vi "NI_USB.vi"() -> ()   [LabVIEW 2014]
doc: "Measure data from NI USB 6343"
uses:
  <vilib>/DAQmx/read.llb/DAQmx Read (Analog 1D Wfm NChan NSamp).vi
  <vilib>/DAQmx/configure/timing.llb/DAQmx Timing (Sample Clock).vi
  <vilib>/DAQmx/create/channels.llb/DAQmx Create Channel (AI-Voltage-Basic).vi
  <resource>/objmgr/daqmx.rc
panel:
  in  "Open PDF":bool
  in  "Help":bool
  out "Realization":dbl caption="Реализация"
  in  "Number of Samples":i16=100 caption="Буффер, от." min=10 max=2000 step=1
  out "init":bool
  in  "Sample Rate":dbl=1000.0 caption="Частота дискретизации, Гц" min=1.0 max=500000.0 step=1.0 format="%#.0f"
  in  "Terminal Config":i32(ring)=10083 caption="Конфигурация подключения" items=["RSE"=10083, "NRSE"=10078, "Differential"=10106]
  in  "Max Voltage":i8=5 caption="Макс. U, B" min=-10 max=10 step=1
  in  "Min Voltage":i8=-5 caption="Мин. U, B" min=-10 max=10 step=1
  in  "Physical Channel":tag="Dev1/ai0" caption="Выбор физических каналов"
  in  "Initialize":bool
  out "Rec":bool
  in  "File Path":path=path "D:/example.tdms"
  in  "Stop Record":bool
  in  "Start Record":bool
  out "WaveGraph":waveform(dbl)[](graph)
  out "Actual Sample Rate":dbl=1000.0 format="%0.2f"
  in  "Shutdown":bool
  in  "Stop Measure":bool
  in  "Start Measure":bool
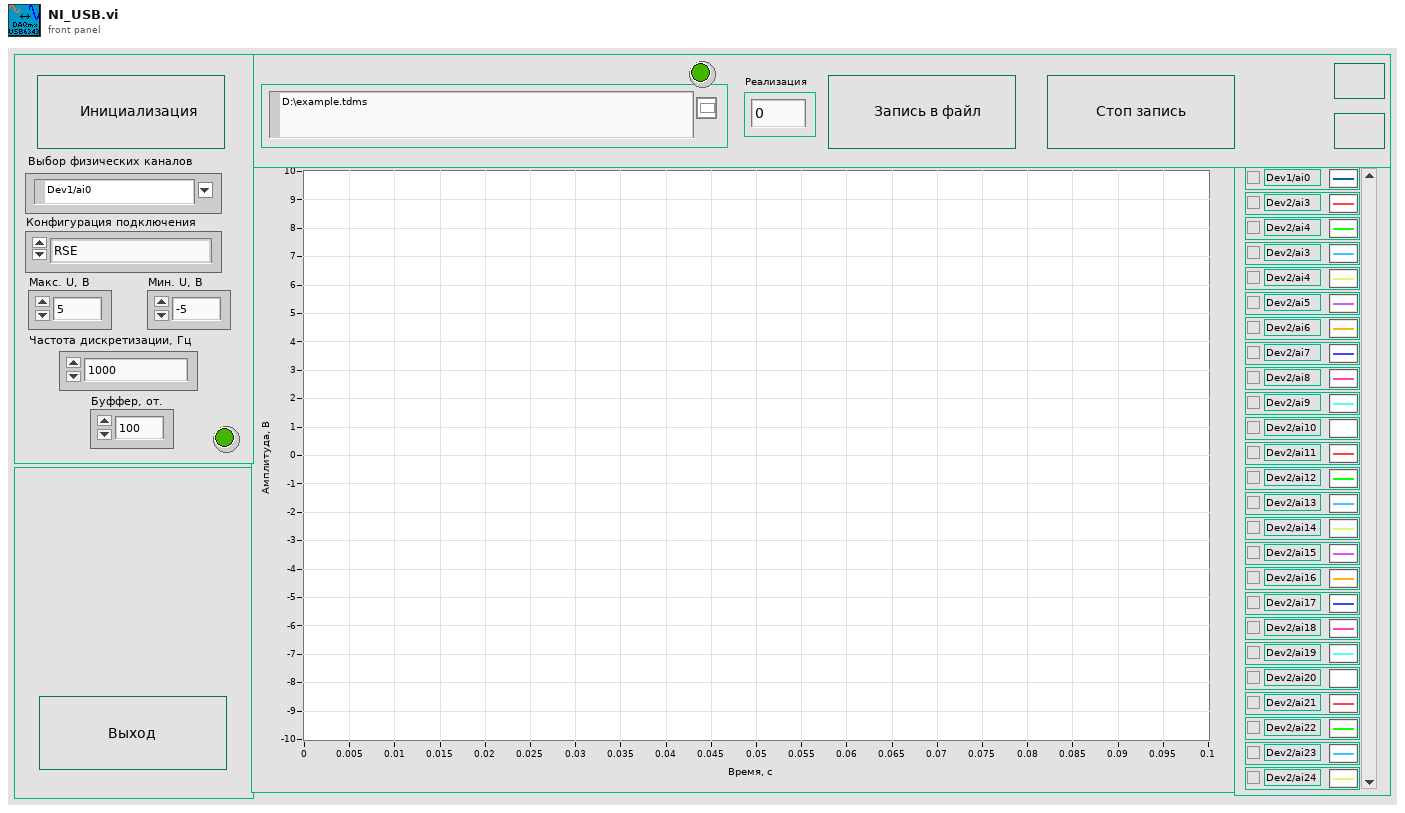
[diagram p1: front panel]
types:
  T1 = enum16{"Initialize", "Start Measure", "Stop Measure", "Start Record", "Stop Record", "Shutdown"}
  T2 = enum32{"invalid app kind", "Development System", "Run Time System", "Student Edition", "Embedded LabVIEW", "Evaluation", "Custom"}
  T3 = enum16{"open", "open or create", "create or replace", "create", "open (read-only)"}
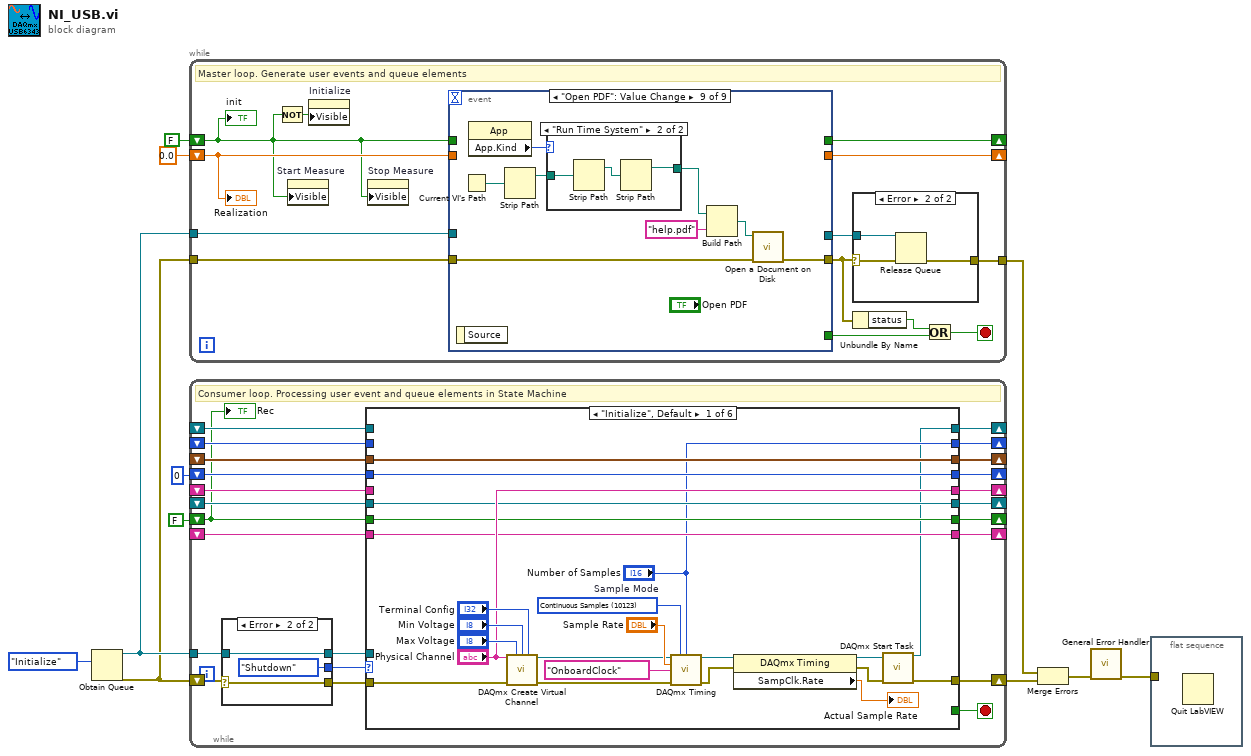
[diagram p0: block diagram]
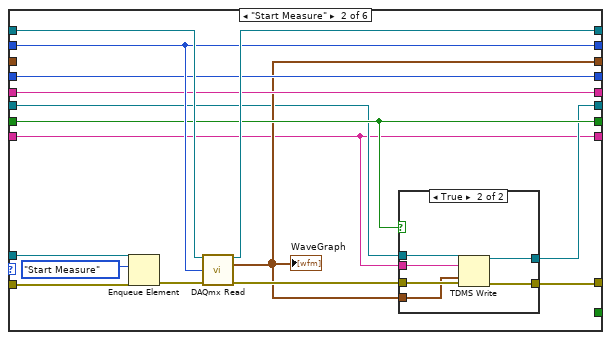
[diagram p2: hidden frame]
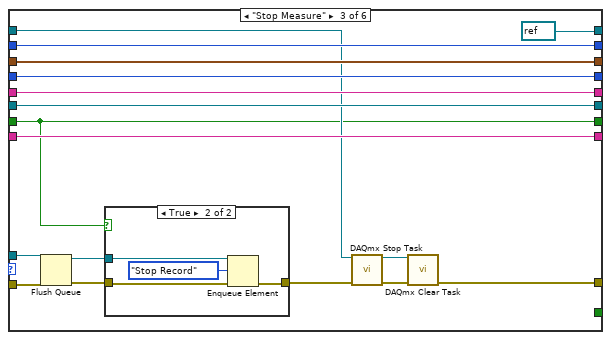
[diagram p4: hidden frame]
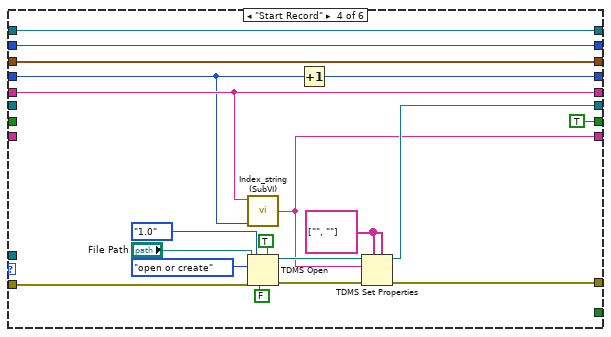
[diagram p6: hidden frame]
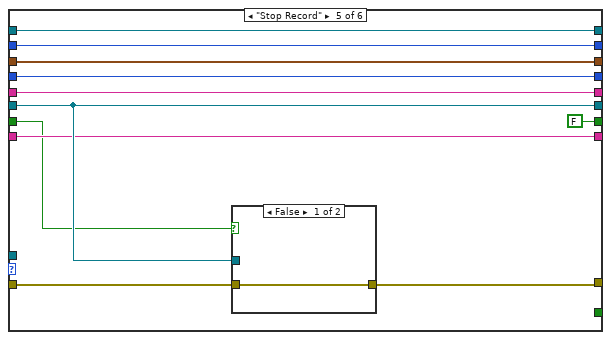
[diagram p7: hidden frame]
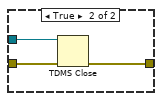
[diagram p8: hidden frame]
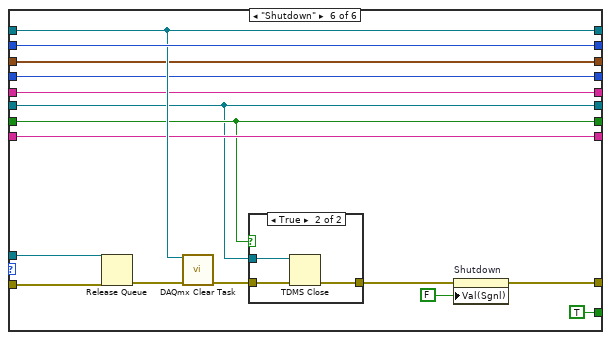
[diagram p9: hidden frame]
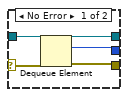
[diagram p11: hidden frame]
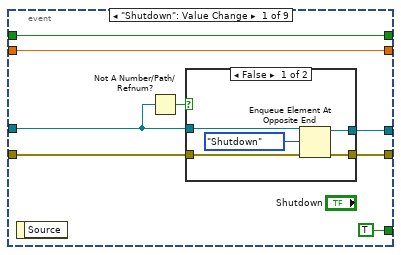
[diagram p13: hidden frame]
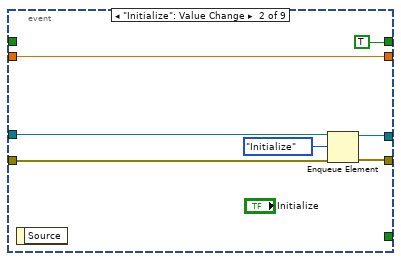
[diagram p15: hidden frame]
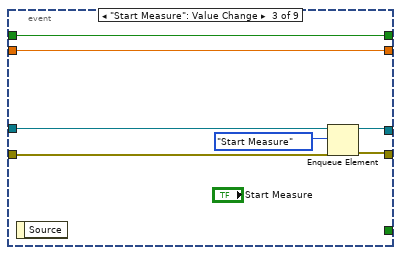
[diagram p16: hidden frame]
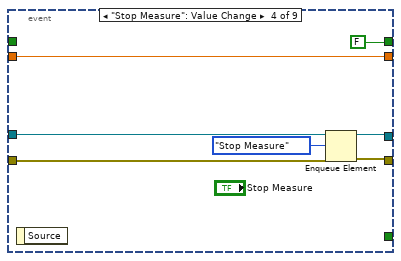
[diagram p17: hidden frame]
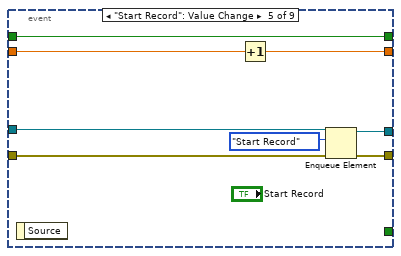
[diagram p18: hidden frame]
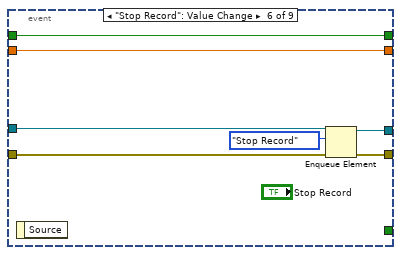
[diagram p19: hidden frame]
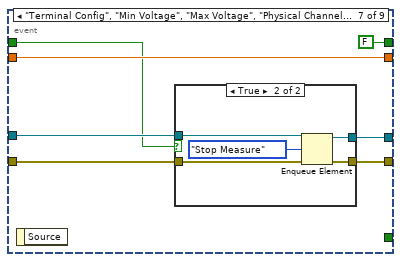
[diagram p20: hidden frame]
diagram:
  n1 = Obtain Queue(element data type=T1."Initialize" ("Enum 2")) -> (queue out=w7:refnum<queue>, error out=w6:errorcluster)  [unwired: 4 in, 1 out]
  n2 = while {
    tunnel: w7 -> [w24]
    tunnel: w6 -> [w23]
    tunnel: [w21] -> w9
    shift-right: [w16] -> _
    shift-left: FALSE -> [w12]
    shift-right: [w15] -> _
    shift-left: 0.0 -> [w14]
    stop <- w17 stop-if-true
    # "Master loop. Generate user events and queue elements"
    n3 = Not(x=w12) -> (.not. x?=w13:bool)
    n4 = property on="Start Measure" class="Bool"("Visible"=w12) -> ()  [unwired: 2 in, 2 out]
    n5 = property on="Initialize" class="Bool"("Visible"=w13) -> ()  [unwired: 2 in, 2 out]
    n6 = property on="Stop Measure" class="Bool"("Visible"=w12) -> ()  [unwired: 2 in, 2 out]
    n7 = event shown="[8] \"Open PDF\": Value Change" {
      selector: _ -> [_ _ _ _ _ _ _ _ _]
      dyn-events: _ -> [_ _ _ _ _ _ _ _ _]
      timeout: _ -> [_ _ _ _ _ _ _ _ _]
      tunnel: [TRUE _ _ _ _ _ _ _ _] -> w18
      tunnel: w24 -> [w35 w47 w56 w61 w70 w77 w83 w97 _]
      tunnel: w23 -> [w36 w50 w57 w64 w71 w78 w84 w98 w106]
      tunnel: [w33 w48 w54 w62 w68 w75 w82 w98 w105] -> w20
      tunnel: [w32 w49 w55 w63 w69 w76 w81 w97 _] -> w22
      tunnel: w12 -> [w31 _ w52 _ w67 w74 w80 w96 _]
      tunnel: [w31 TRUE w52 FALSE w67 w74 FALSE w96 _] -> w16
      tunnel: w14 -> [w30 w45 w51 w59 w66 w73 w85 w95 _]
      tunnel: [w30 w45 w51 w59 w65 w73 w85 w95 _] -> w15
      event "Shutdown": Value Change {
        n8 = event-data() -> ()  [unwired: 1 in, 1 out]
        n9 = Not A Number/Path/Refnum?(number/path/refnum=w35) -> (NaN/Path/Refnum?=w34:bool)
        n10 = case shown="False" w34 {
          tunnel: w35 -> [w41 w42]
          tunnel: w36 -> [w40 w43]
          tunnel: [w39 w43] -> w33
          tunnel: [w38 w42] -> w32
          frame False {
            n11 = Enqueue Element At Opposite End(queue=w41, element=T1."Shutdown" ("Enum 2"), error in (no error)=w40) -> (queue out=w38:refnum<queue>, error out=w39:errorcluster)  [unwired: 1 in, 1 out]
          }
          frame True {
          }
        }
      }
      event "Initialize": Value Change {
        n12 = event-data() -> ()  [unwired: 1 in, 1 out]
        n13 = Enqueue Element(queue=w47, element=T1."Initialize" ("Enum 2"), error in (no error)=w50) -> (queue out=w49:refnum<queue>, error out=w48:errorcluster)  [unwired: 1 in, 1 out]
      }
      event "Start Measure": Value Change {
        n14 = event-data() -> ()  [unwired: 1 in, 1 out]
        n15 = Enqueue Element(queue=w56, element=T1."Start Measure" ("Enum 2"), error in (no error)=w57) -> (queue out=w55:refnum<queue>, error out=w54:errorcluster)  [unwired: 1 in, 1 out]
      }
      event "Stop Measure": Value Change {
        n16 = event-data() -> ()  [unwired: 1 in, 1 out]
        n17 = Enqueue Element(queue=w61, element=T1."Stop Measure" ("Enum 2"), error in (no error)=w64) -> (queue out=w63:refnum<queue>, error out=w62:errorcluster)  [unwired: 1 in, 1 out]
      }
      event "Start Record": Value Change {
        n18 = event-data() -> ()  [unwired: 1 in, 1 out]
        n19 = Increment(x=w66) -> (x+1=w65:dbl)
        n20 = Enqueue Element(queue=w70, element=T1."Start Record" ("Enum 2"), error in (no error)=w71) -> (queue out=w69:refnum<queue>, error out=w68:errorcluster)  [unwired: 1 in, 1 out]
      }
      event "Stop Record": Value Change {
        n21 = event-data() -> ()  [unwired: 1 in, 1 out]
        n22 = Enqueue Element(queue=w77, element=T1."Stop Record" ("Enum 2"), error in (no error)=w78) -> (queue out=w76:refnum<queue>, error out=w75:errorcluster)  [unwired: 1 in, 1 out]
      }
      event "Terminal Config", "Min Voltage", "Max Voltage", "Physical Channel", "Sample Rate", "Number of Samples": Value Change {
        n23 = event-data() -> ()  [unwired: 1 in, 1 out]
        n24 = case shown="True" w80 {
          tunnel: w84 -> [w87 w92]
          tunnel: w83 -> [w88 w91]
          tunnel: [w87 w90] -> w82
          tunnel: [w88 w89] -> w81
          frame False {
          }
          frame True {
            n25 = Enqueue Element(queue=w91, element=T1."Stop Measure" ("Enum 2"), error in (no error)=w92) -> (queue out=w89:refnum<queue>, error out=w90:errorcluster)  [unwired: 1 in, 1 out]
          }
        }
      }
      event "Help": Value Change {
        n26 = event-data() -> ()  [unwired: 1 in, 1 out]
        n27 = Control Help Window(1:TRUE ("Show")) -> ()  [unwired: 1 in]
      }
      event "Open PDF": Value Change {
        n28 = event-data() -> ()  [unwired: 1 in, 1 out]
        n29 = Current VI's Path() -> (path=w101:path)
        n30 = property class="App"() -> ("App.Kind"=w102:T2)  [unwired: 2 in, 2 out]
        n31 = Strip Path(path=w101) -> (stripped path=w103:path)  [unwired: 1 out]
        n32 = case shown="\"Run Time System\"" w102 {
          tunnel: w103 -> [w107 w110]
          tunnel: [w107 w109] -> w104
          frame Default {
          }
          frame "Run Time System" {
            n33 = Strip Path(path=w110) -> (stripped path=w108:path)  [unwired: 1 out]
            n34 = Strip Path(path=w108) -> (stripped path=w109:path)  [unwired: 1 out]
          }
        }
        n35 = Build Path(base path=w104, name or relative path="help.pdf") -> (appended path=w99:path)
        n36 = call <vilib>:"Open a Document on Disk.vi"("error in (no error)"=w106, "document path"=w99) -> ("error out"=w105:errorcluster)  [unwired: 5 in]
      }
    }
    n37 = case shown="Error" w20 {
      selector: w20 -> [w25 w28]
      tunnel: w22 -> [_ w27]
      tunnel: [w25 w26] -> w21
      frame No Error {
      }
      frame Error {
        n38 = Release Queue(queue=w27, error in (no error)=w28) -> (error out=w26:errorcluster)  [unwired: 1 in, 2 out]
      }
    }
    n39 = Unbundle By Name(w20) -> ("status"=w19:bool)
    n40 = Or(x=w19, y=w18) -> (x .or. y?=w17:bool)
    "init" <- w12
    "Realization" <- w14
  }
  n41 = while {
    tunnel: w7 -> [w132]
    shift-right: [w127] -> w10
    shift-left: w6 -> [w133]
    shift-right: [w126] -> _
    shift-left: _ -> [w125]
    shift-right: [w124] -> _
    shift-left: _ -> [w123]
    shift-right: [w122] -> _
    shift-left: _ -> [w121]
    shift-right: [w119] -> _
    shift-left: 0 -> [w120]
    shift-right: [w118] -> _
    shift-left: _ -> [w117]
    shift-right: [w116] -> _
    shift-left: _ -> [w115]
    shift-right: [w114] -> _
    shift-left: FALSE -> [w111]
    shift-right: [w113] -> _
    shift-left: _ -> [w112]
    stop <- w128 stop-if-true
    # "Consumer loop. Processing user event and queue elements in State Machine"
    n42 = case shown="Error" w133 {
      selector: w133 -> [w261 w263]
      tunnel: [w259 T1."Shutdown" ("Enum 2")] -> w131
      tunnel: [w258 w263] -> w130
      tunnel: [w257 w262] -> w129
      tunnel: w132 -> [w260 w262]
      frame No Error {
        n43 = Dequeue Element(queue=w260, error in (no error)=w261) -> (queue out=w257:refnum<queue>, element=w259:T1, error out=w258:errorcluster)  [unwired: 1 in, 1 out]
      }
      frame Error {
      }
    }
    n44 = case shown="\"Initialize\", Default" w131 {
      tunnel: w130 -> [w138 w169 w193 w205 w227 w252]
      tunnel: w129 -> [_ w167 w192 _ _ w251]
      tunnel: [_ _ _ _ _ TRUE] -> w128
      tunnel: [w144 w163 w195 w207 w226 w249] -> w127
      tunnel: [w134 w171 refnum<k21> refnum ("task out") w210 w232 w246] -> w126
      tunnel: w125 -> [_ w172 w186 w210 w232 w246]
      tunnel: ["Number of Samples" w170 w197 w221 w231 w248] -> w124
      tunnel: w123 -> [_ w170 w197 w221 w231 w248]
      tunnel: [w142 w160 w191 w220 w230 w245] -> w122
      tunnel: w121 -> [w142 _ w191 w220 w230 w245]
      tunnel: w120 -> [w141 w165 w190 w208 w229 w244]
      tunnel: [w141 w165 w190 w211 w229 w244] -> w119
      tunnel: ["Physical Channel" w164 w189 w209 w228 w243] -> w118
      tunnel: w117 -> [_ w164 w189 w209 w228 w243]
      tunnel: [w139 w158 w188 w206 w225 w238] -> w116
      tunnel: w115 -> [w139 w159 w188 _ w225 w238]
      tunnel: [w137 w161 w184 TRUE FALSE w239] -> w114
      tunnel: w111 -> [w137 w161 w184 _ w222 w239]
      tunnel: [w136 w157 w187 w203 w223 w242] -> w113
      tunnel: w112 -> [w136 w157 w187 _ w223 w242]
      frame "Initialize", Default {
        w148 = 10123 items=["Finite Samples"=10178, "Continuous Samples"=10123, "Hardware Timed Single Point"=12522]  # Sample Mode
        n45 = call-poly <vilib>:"DAQmx Create Virtual Channel.vi"("maximum value"="Max Voltage", "minimum value"="Min Voltage", "input terminal configuration"="Terminal Config", "physical channels"="Physical Channel", "error in"=w138) -> ("task out"=w150:refnum<k21>, "error out"=w149:errorcluster)  [unwired: 9 in]
        n46 = call-poly <vilib>:"DAQmx Timing.vi"("task/channels in"=w150, "sample mode"=w148, "samples per channel"="Number of Samples", "rate"="Sample Rate", "source"=tag "OnboardClock", "error in"=w149) -> ("task out"=w146:refnum<k21>, "error out"=w147:errorcluster)  [unwired: 8 in]
        n47 = property class="DAQmx Timing"(reference=w146, error in=w147) -> (reference out=w143:refnum<k21>, error out=w145:errorcluster, "SampClk.Rate"=→"Actual Sample Rate":dbl)
        n48 = call <vilib>:"DAQmx Start Task.vi"("task/channels in"=w143, "error in"=w145) -> ("task out"=w134:refnum<k21>, "error out"=w144:errorcluster)  [unwired: 12 in]
      }
      frame "Start Measure" {
        n49 = Enqueue Element(queue=w167, element=T1."Start Measure" ("Enum 2"), error in (no error)=w169) -> (error out=w168:errorcluster)  [unwired: 1 in, 2 out]
        n50 = call-poly <vilib>:"DAQmx Read.vi"("task/channels in"=w172, "number of samples per channel"=w170, "error in"=w168) -> ("task out"=w171:refnum<k21>, "data"=w160:waveform(dbl)[], "error out"=w162:errorcluster)  [unwired: 10 in]
        "WaveGraph" <- w160
        n51 = case shown="True" w161 {
          tunnel: [w174 w180] -> w163
          tunnel: w162 -> [w174 w179]
          tunnel: w157 -> [_ w176]
          tunnel: w160 -> [_ w178]
          tunnel: w159 -> [w173 w177]
          tunnel: [w173 w175] -> w158
          frame False {
          }
          frame True {
            n52 = TDMS Write(0:w177, 5:w176, 9:w178, 11:w179) -> (4:w175:refnum<k34>, 15:w180:errorcluster)  [unwired: 2 in, 2 out]
          }
        }
      }
      frame "Stop Measure" {
        n53 = Flush Queue(queue=w192, error in (no error)=w193) -> (queue out=w183:refnum<queue>, error out=w182:errorcluster)  [unwired: 1 out]
        n54 = case shown="True" w184 {
          tunnel: w183 -> [_ w199]
          tunnel: w182 -> [w198 w201]
          tunnel: [w198 w200] -> w181
          frame False {
          }
          frame True {
            n55 = Enqueue Element(queue=w199, element=T1."Stop Record" ("Enum 2"), error in (no error)=w201) -> (error out=w200:errorcluster)  [unwired: 1 in, 2 out]
          }
        }
        n56 = call <vilib>:"DAQmx Stop Task.vi"("task/channels in"=w186, "error in"=w181) -> ("task out"=w194:refnum<k21>, "error out"=w196:errorcluster)  [unwired: 12 in]
        n57 = call <vilib>:"DAQmx Clear Task.vi"("task in"=w194, "error in"=w196) -> ("error out"=w195:errorcluster)  [unwired: 13 in]
      }
      frame "Start Record" {
        w219 = string[] ["", ""] ("property names")
        n58 = call "Index_string (SubVI).vi"("Index(0..X)"=w208, "Physical Channel"=w209) -> ("Result"=w203:string)  [unwired: 2 in]
        n59 = TDMS Open(5:TRUE ("create index file? (T)"), 6:FALSE ("disable buffering? (T)"), 7:enum16{"1.0", "2.0"}."1.0" ("file format version (2.0)"), 8:w205, 10:T3."open or create" ("operation (0:open)"), 11:"File Path") -> (0:w215:errorcluster, 3:w214:refnum<k34>)  [unwired: 1 in]
        n60 = Increment(x=w208) -> (x+1=w211:i32)
        n61 = TDMS Set Properties(5:w219, 7:w219, 8:w215, 10:w203, 11:w214) -> (0:w207:errorcluster, 3:w206:refnum<k34>)  [unwired: 1 in, 2 out]
      }
      frame "Stop Record" {
        n62 = case shown="False" w222 {
          tunnel: w227 -> [w233 w236]
          tunnel: [w233 w235] -> w226
          tunnel: w225 -> [_ w234]
          frame False {
          }
          frame True {
            n63 = TDMS Close(8:w236, 11:w234) -> (0:w235:errorcluster)  [unwired: 1 out]
          }
        }
      }
      frame "Shutdown" {
        n64 = Release Queue(queue=w251, error in (no error)=w252) -> (error out=w247:errorcluster)  [unwired: 1 in, 2 out]
        n65 = call <vilib>:"DAQmx Clear Task.vi"("task in"=w246, "error in"=w247) -> ("error out"=w241:errorcluster)  [unwired: 13 in]
        n66 = case shown="True" w239 {
          tunnel: w241 -> [w253 w256]
          tunnel: [w253 w255] -> w240
          tunnel: w238 -> [_ w254]
          frame False {
          }
          frame True {
            n67 = TDMS Close(8:w256, 11:w254) -> (0:w255:errorcluster)  [unwired: 1 out]
          }
        }
        n68 = property on="Shutdown" class="Bool (strict)"(error in=w240, "Val(Sgnl)"=FALSE) -> (error out=w249:errorcluster)  [unwired: 1 in, 1 out]
      }
    }
    "Rec" <- w111
  }
  n69 = Merge Errors(w9, w10) -> (w8:errorcluster)
  n70 = call <vilib>:"General Error Handler.vi"("error in (no error)"=w8) -> ("error out"=w1:errorcluster)  [unwired: 10 in, 4 out]
  n71 = flat-sequence {
    tunnel: w1 -> [_]
    frame #0 {
      n72 = Quit LabVIEW() -> ()  [unwired: 1 in]
    }
  }
